vi "Test_Observe_ModelPublication_OK.vi"(8 "error in (no error)":errorcluster, 11 "TestObservation In":refnum<class "TestObservation.lvclass">) -> (0 "error out":errorcluster, 3 "TestObservation Out":refnum<class "TestObservation.lvclass">)   [LabVIEW 2017, in "TestObservation.lvlib" / "TestObservation.lvclass"]
uses:
  TestObservation.lvclass
  PublishingModel/PublishingModel.lvclass
  C:/Git/mva-framework/Framework/IModel/IModel/IModel.lvclass
  Source/Framework/Mediator/Mediator/Mediator.lvclass
  C:/Git/mva-framework/Framework/IMediator/IMediator/IMediator.lvclass
  Source/Framework/IViewModel/IViewModel/IViewModel.lvclass/IViewModel.ctl
  Source/Framework/IViewManager/IViewManager Messages/Launch Nested Views Msg/Launch Nested Views Msg.lvclass/Launch Nested Views Msg.ctl
  Source/Framework/IViewManager/IViewManager/IViewManager.lvclass/IViewManager.ctl
  <vilib>/ActorFramework/Message Enqueuer/Message Enqueuer.lvclass/Message Enqueuer.ctl
  Source/Framework/IViewManager/IViewManager Messages/Launch Nested Views Msg/Pack Launch Nested Views Msg.vi
  Source/Framework/IViewManager/IViewManager/Write Startup Launch Nested Views Msg.vi
  <vilib>/ActorFramework/Message Enqueuer/Enqueue.vi
  ObservingViewable/ObservingViewable.lvclass
  C:/Git/mva-framework/Framework/IViewable/IViewable/IViewable.lvclass
  ObservingViewModel/ObservingViewModel.lvclass
  C:/Git/mva-framework/Framework/IViewModel/IViewModel/IViewModel.lvclass
  C:/Program Files (x86)/National Instruments/LabVIEW 2017/vi.lib/ActorFramework/Actor/Actor.lvclass
  Source/Framework/IViewModel/IViewModel/IViewModel.lvclass
  C:/Git/mva-framework/Framework/IViewManager/IViewManager/IViewManager.lvclass
  <vilib>/ActorFramework/Stop Msg/Stop Msg.lvclass
  C:/Program Files (x86)/National Instruments/LabVIEW 2017/vi.lib/ActorFramework/Message/Message.lvclass
  <vilib>/ActorFramework/Message Priority Queue/Priority Enqueue.vi
  Source/Framework/IViewable/IApplicationStyle/IApplicationStyle.lvclass
  Source/Framework/IViewManager/IViewManager Messages/Launch Nested Views Msg/Launch Nested Views Msg.lvclass
  <vilib>/addons/_JKI Toolkits/VI Tester/TestCase.llb/TestCase.lvclass
  <vilib>/ActorFramework/Actor/Actor.lvclass
  C:/Program Files (x86)/National Instruments/LabVIEW 2017/vi.lib/addons/_JKI Toolkits/VI Tester/TestCase.llb/TestCase.lvclass
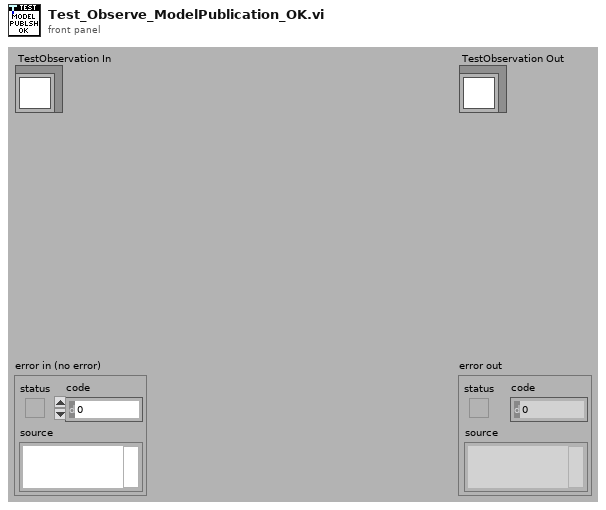
[diagram p1: front panel]
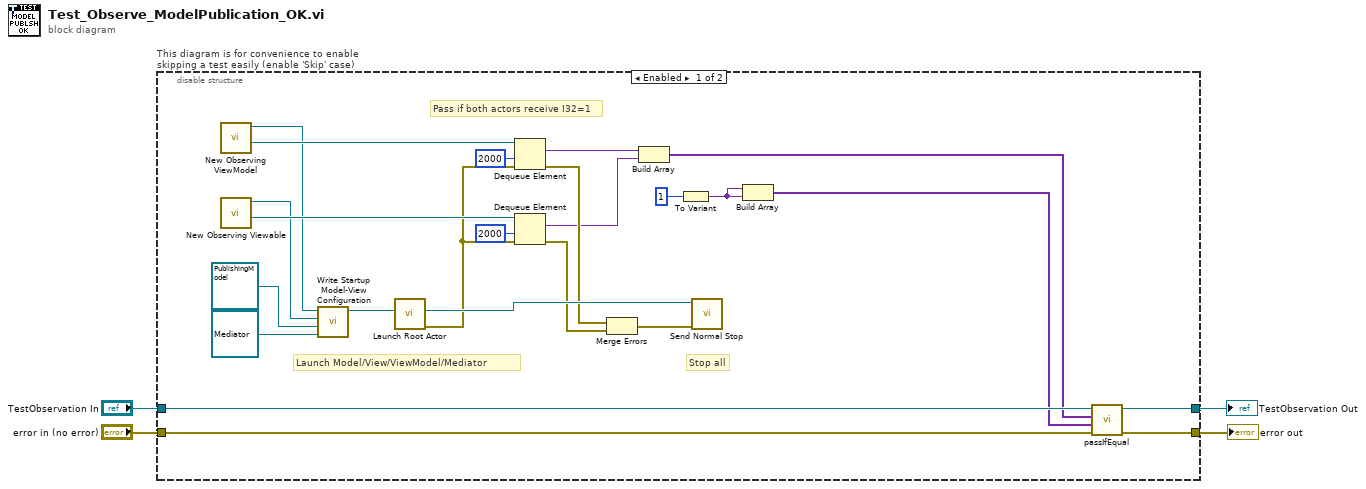
[diagram p0: block diagram]
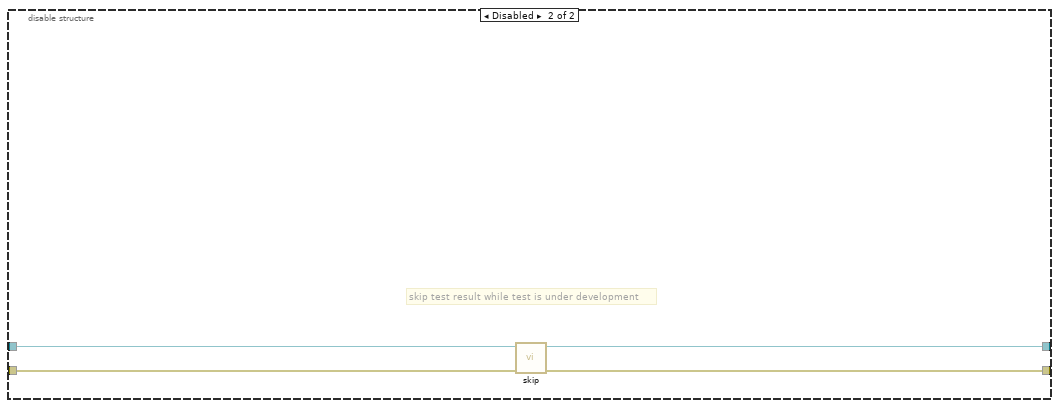
[diagram p2: hidden frame]
diagram:
  n1 = disable-structure "This diagram is for convenience to enable skipping a test easily (enable 'Skip' case)" shown="Enabled" {
    disable-tunnel: "TestObservation In" -> [w28 w32]
    disable-tunnel: [w27 w30] -> w1
    disable-tunnel: [w26 w31] -> w3
    disable-tunnel: "error in (no error)" -> [w25 w29]
    frame Enabled {
      # "Stop all"
      # "Launch Model/View/ViewModel/Mediator"
      # "Pass if both actors receive I32=1"
      n2 = call "New Observing ViewModel.vi"() -> ("Test Reply Queue"=w15:refnum<queue>, "ObservingViewModel Out"=w6:refnum<class "ObservingViewModel.lvclass">)  [unwired: 10 in]
      n3 = call "New Observing Viewable.vi"() -> ("Test Reply Queue"=w21:refnum<queue>, "ObservingViewable out"=w7:refnum<class "ObservingViewable.lvclass">)  [unwired: 10 in]
      n4 = call "Write Startup Model-View Configuration.vi"("Mediator Type"=refnum<class "Mediator.lvclass"> refnum ("Mediator.lvlib:Mediator.lvclass"), "Model Type"=refnum<class "PublishingModel.lvclass"> refnum ("PublishingModel.lvclass"), "Startup View Configuration"=w7, "IViewModel In"=w6) -> ("IViewModel Out"=w22:refnum<class "ObservingViewModel.lvclass">)  [unwired: 7 in]
      n5 = call <vilib>:"Launch Root Actor.vi"("Actor"=w22) -> ("error out"=w5:errorcluster, "Actor's Enqueuer"=w19:refnum<class "Message Enqueuer.lvclass">)  [unwired: 9 in]
      n6 = Dequeue Element(queue=w15, timeout in ms (-1)=2000, error in (no error)=w5) -> (element=w12:variant, error out=w13:errorcluster)  [unwired: 2 out]
      n7 = Dequeue Element(queue=w21, timeout in ms (-1)=2000, error in (no error)=w5) -> (element=w11:variant, error out=w18:errorcluster)  [unwired: 2 out]
      n8 = Merge Errors(w13, w18) -> (w14:errorcluster)
      n9 = Build Array(w12, w11) -> (w10:variant[])
      n10 = To Variant(anything=1) -> (Variant=w8:variant)
      n11 = call <vilib>:"Send Normal Stop.vi"("error in (no error)"=w14, "Message Enqueuer"=w19) -> ()  [unwired: 9 in, 1 out]
      n12 = Build Array(w8, w8) -> (w9:variant[])
      n13 = call-dynamic "passIfEqual.vi"("error in (no error)"=w25, "y"=w9, "x"=w10, "TestCase in"=w28) -> ("error out"=w26:errorcluster, "TestCase out"=w27:refnum<class "TestObservation.lvclass">)  [unwired: 6 in]
    }
    frame Disabled {
      # "skip test result while test is under development"
      n14 = call <vilib>:"skip.vi"("error in (no error)"=w29, "TestCase in"=w32) -> ("error out"=w31:errorcluster, "TestCase out"=w30:refnum<class "TestObservation.lvclass">)  [unwired: 8 in]
    }
  }
  "error out" <- w3
  "TestObservation Out" <- w1
